vi "StepperControl.vi"(10 "speed":u32(knob) scale=1.0..10.0, 11 "sweep angle\n(9 degree increments work best)":i32) -> ()   [LabVIEW 2014]
uses:
  StepperData.vi
  globe stop.vi
panel:
  # "Stepper Motor Control"
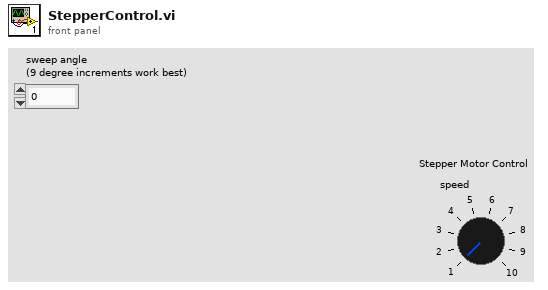
[diagram p1: front panel]
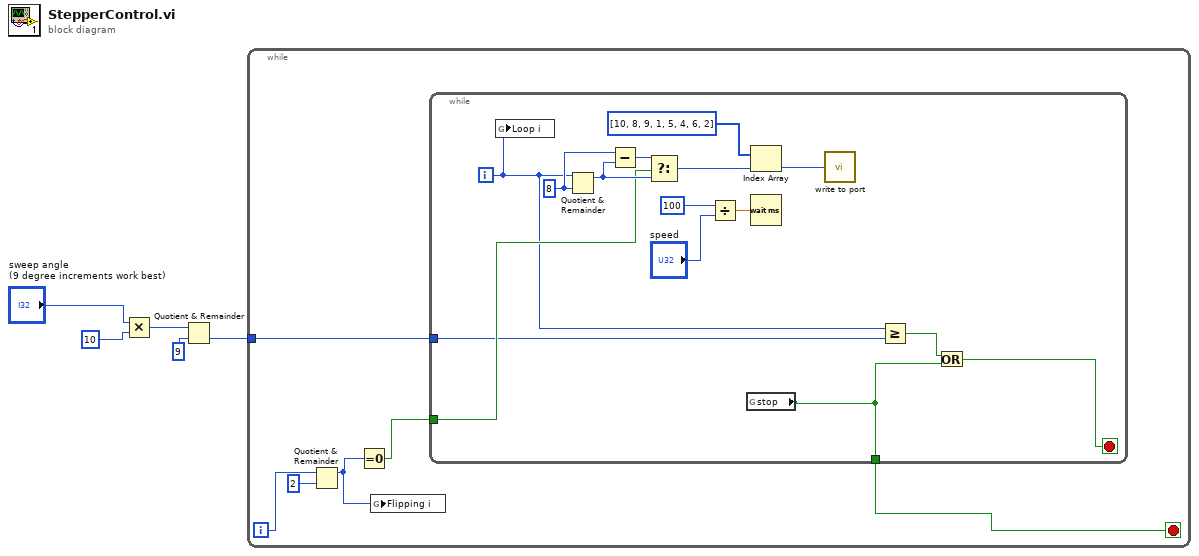
[diagram p0: block diagram]
diagram:
  n1 = Multiply(x="sweep angle\n(9 degree increments work best)", y=10) -> (x*y=w5:i32)
  n2 = Quotient & Remainder(x=w5, y=9) -> (floor(x/y)=w1:i32)  [unwired: 1 out]
  n3 = while {
    tunnel: w1 -> [w9]
    i -> [w7]
    stop <- w10 stop-if-true
    n4 = Quotient & Remainder(x=w7, y=2) -> (x-y*floor(x/y)=w6:i32)  [unwired: 1 out]
    n5 = Equal To 0?(x=w6) -> (x = 0?=w8:bool)
    n6 = global write "StepperData.vi" "Flipping i"(w6) -> ()
    n7 = while {
      tunnel: w8 -> [w17]
      tunnel: [w12] -> w10
      tunnel: w9 -> [w15]
      i -> [w13]
      stop <- w16 stop-if-true
      w22 = 8 ("y")
      n8 = global write "StepperData.vi" "Loop i"(w13) -> ()
      n9 = Quotient & Remainder(x=w13, y=w22) -> (x-y*floor(x/y)=w21:i32)  [unwired: 1 out]
      n10 = Subtract(x=w22, y=w21) -> (x-y=w23:i32)
      n11 = Select(t=w23, s=w17, f=w21) -> (s? t:f=w24:i32)
      n12 = Divide(x=u32 100, y="speed") -> (x/y=w20:dbl)
      n13 = global read "globe stop.vi" "stop"() -> (w12:bool)
      n14 = Index Array(array=i32[] [10, 8, 9, 1, 5, 4, 6, 2], index=w24) -> (element=w26:i32)
      n15 = Wait (ms)(milliseconds to wait=w20) -> ()  [unwired: 1 out]
      n16 = call "write to port.vi"("number to write to port"=w26) -> ()
      n17 = Greater Or Equal?(x=w13, y=w15) -> (x >= y?=w14:bool)
      n18 = Or(x=w14, y=w12) -> (x .or. y?=w16:bool)
    }
  }
